vi "Display Input (String) Popup.vi"(6 "Theme":refnum<class "Theme.lvclass">, 7 "Display Style":u32(ring) items=["Normal Display", "'\\' Codes Display", "Password Display", "Hex Display"], 8 "error in":errorcluster, 9 "Default Input":string, 10 "Message":string, 11 "Graphic":T1="info") -> (0 "error out":errorcluster, 1 "Input Value":string)   [LabVIEW 2021, in "Pop-Up.lvlib" / "Input (String).lvclass"]
doc: "The input (String) popup will display information to the user and wait for the operator to enter a value and click the button.\n\n<b>Note:</b> The function <b>Close Pop-Up (String).vi</b> can be used to send a value when closing this dialog. Otherwise, use Close Pop-Up.vi to close it early.\n\nInputs:\n-Graphic [typedef combobox] - Image (PNG) for Graphic for Popup\n-Message [String] - String Variable to populate Display\n-Theme [lvclass] - the theme for the style of the popup\n-Default Input [string] - default value for the prompt\n\nOutputs\n-Input Value [String] - the user's entered data\n\n<b>Code Developed By:</b>\nDaniel Coons\nTechnology Service Corporation\n1983 S Liberty Drive\nBloomington, IN 47403\nPhone: 812 558-7100\ndaniel.coons@tsc.com\nwww.tsc.com/atcs"
uses:
  Input (String).lvclass
  Graphics.ctl
  Theme/Theme.lvclass
  Input (String).lvclass/Input (String).ctl
  Pop-Up.lvlib
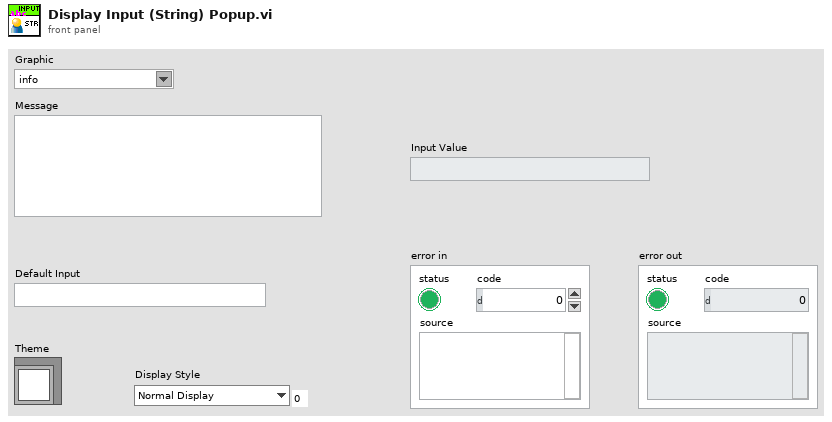
[diagram p1: front panel]
types:
  T1 = typedef "Pop-Up.lvlib/Graphics.ctl" = string
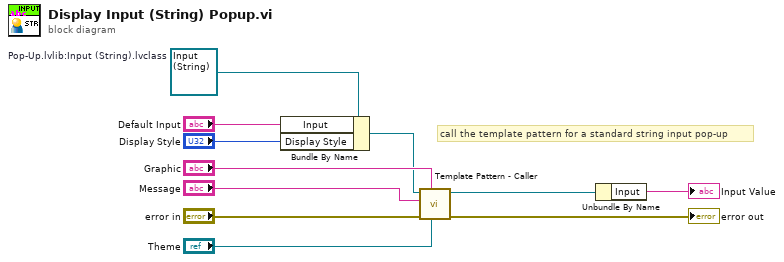
[diagram p0: block diagram]
diagram:
  w7 = refnum<class "Input (String).lvclass"> refnum  # Pop-Up.lvlib:Input (String).lvclass
  # "call the template pattern for a standard string input pop-up"
  n1 = Bundle By Name(cluster=w7, "Input"="Default Input", "Display Style"="Display Style") -> (w4:refnum<class "Input (String).lvclass">)
  n2 = call-dynamic "Template Pattern - Caller.vi"("Theme"="Theme", "standard"="Graphic", "error in (no error)"="error in", "Message"="Message", "Pop-Up in"=w4) -> ("error out"=→"error out":errorcluster, "Pop-Up out"=w5:refnum<class "Input (String).lvclass">)  [unwired: 5 in]
  n3 = Unbundle By Name(w5) -> ("Input"=→"Input Value":string)
